vi "SessionBank.vi"(7 "Action (Get)":T1=enum."Get", 8 "error in (no error)":errorcluster, 11 "PythonSession in":refnum<class "PythonSession.lvclass">) -> (0 "error out":errorcluster, 3 "PythonSession out":refnum<class "PythonSession.lvclass">)   [LabVIEW 2022 SP3, in "PythonWrapper.lvlib" / "PythonSession.lvclass"]
uses:
  PythonSession.lvclass
  _BankAction.ctl
  PythonSession.lvclass/PythonSession.ctl
  _BankData.ctl
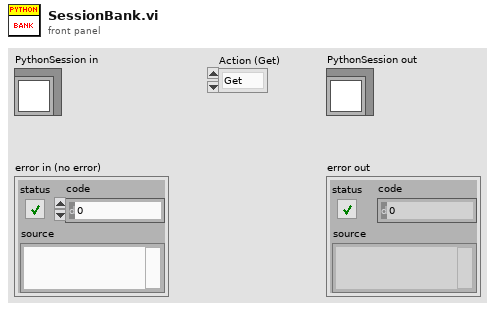
[diagram p1: front panel]
types:
  T1 = typedef "PythonWrapper.lvlib/PythonSession.lvclass/_BankAction.ctl" = enum16{"Add", "Get", "Remove"}
  T2 = typedef "PythonWrapper.lvlib/PythonSession.lvclass/_BankData.ctl" = cluster{"PythonSession":refnum<k35>, "ReferenceCounter":u32}
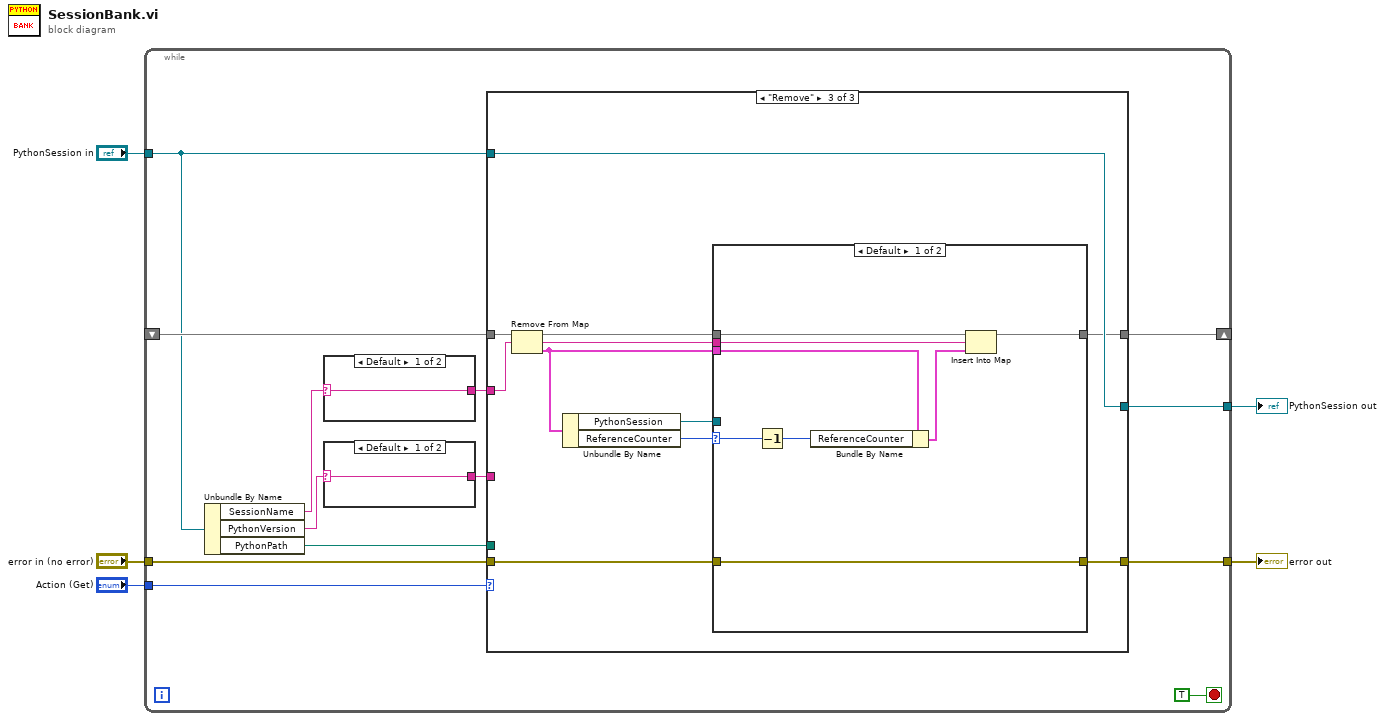
[diagram p0: block diagram]
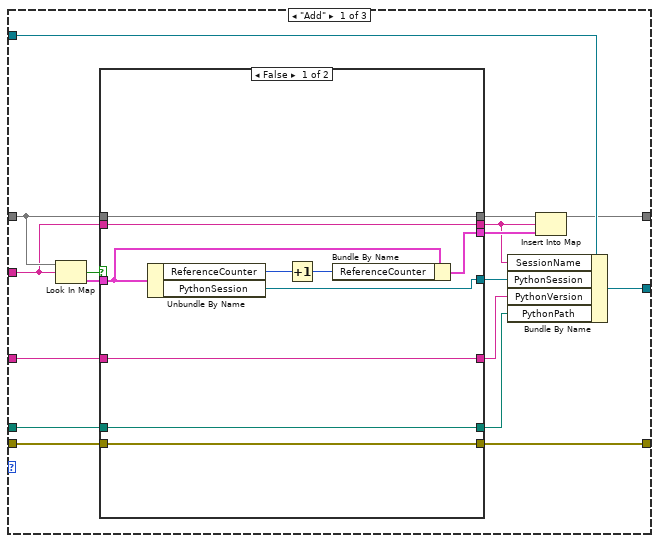
[diagram p2: hidden frame]
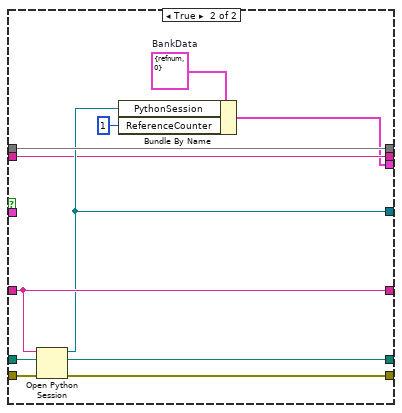
[diagram p3: hidden frame]
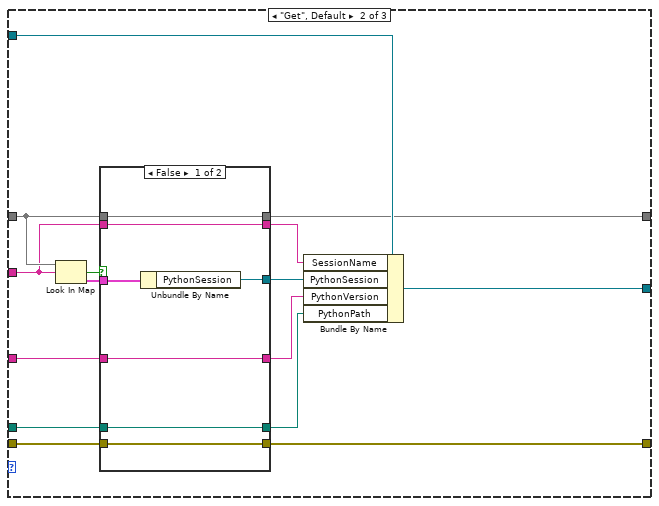
[diagram p4: hidden frame]
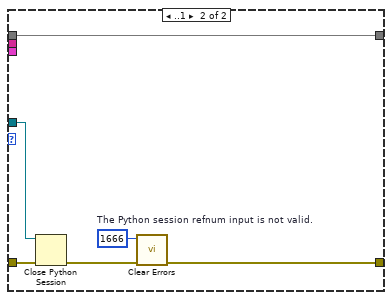
[diagram p6: hidden frame]
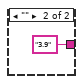
[diagram p7: hidden frame]
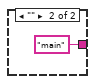
[diagram p8: hidden frame]
diagram:
  n1 = while {
    tunnel: "Action (Get)" -> [w17]
    shift-right: [w13] -> _
    shift-left: _ -> [w16]
    tunnel: "PythonSession in" -> [w10]
    tunnel: "error in (no error)" -> [w15]
    tunnel: [w14] -> w2
    tunnel: [w12] -> w1
    stop <- TRUE stop-if-true
    n2 = Unbundle By Name(w10) -> ("SessionName"=w9:string, "PythonVersion"=w7:string, "PythonPath"=w11:path)
    n3 = case shown="Default" w9 {
      selector: w9 -> [w106 _]
      tunnel: [w106 "main"] -> w8
      frame Default {
      }
      frame "" {
      }
    }
    n4 = case shown="Default" w7 {
      selector: w7 -> [w104 _]
      tunnel: [w104 "3.9"] -> w6
      frame Default {
      }
      frame "" {
      }
    }
    n5 = case shown="\"Remove\"" w17 {
      tunnel: w16 -> [w34 w69 w89]
      tunnel: w15 -> [w33 w68 w88]
      tunnel: [w32 w67 w80] -> w14
      tunnel: w6 -> [w31 w66 _]
      tunnel: w11 -> [w30 w65 _]
      tunnel: [w21 w56 w83] -> w13
      tunnel: [w27 w62 w87] -> w12
      tunnel: w10 -> [w26 w61 w87]
      tunnel: w8 -> [w25 w60 w82]
      frame "Add" {
        n6 = Look In Map(map=w34, key=w25) -> (key not found?=w35:bool, value=w29:T2)  [unwired: 1 in]
        n7 = case shown="False" w35 {
          tunnel: w34 -> [w41 w55]
          tunnel: w25 -> [w40 w48]
          tunnel: w33 -> [w45 w54]
          tunnel: [w45 w53] -> w32
          tunnel: w31 -> [w43 w51]
          tunnel: w30 -> [w44 w52]
          tunnel: [w41 w55] -> w22
          tunnel: w29 -> [w39 _]
          tunnel: [w42 w49] -> w28
          tunnel: [w44 w52] -> w24
          tunnel: [w43 w51] -> w23
          tunnel: [w40 w48] -> w19
          tunnel: [w37 w47] -> w20
          frame False {
            n8 = Unbundle By Name(w39) -> ("ReferenceCounter"=w36:u32, "PythonSession"=w42:refnum<k35>)
            n9 = Increment(x=w36) -> (x+1=w38:u32)
            n10 = Bundle By Name(cluster=w39, "ReferenceCounter"=w38) -> (w37:T2)
          }
          frame True {
            w50 = T2 {"PythonSession"=refnum, "ReferenceCounter"=0}  # BankData
            n11 = Open Python Session(python version=w51, python path=w52, 3:w54) -> (session out=w49:refnum<k35>, error out=w53:errorcluster)
            n12 = Bundle By Name(cluster=w50, "PythonSession"=w49, "ReferenceCounter"=u32 1) -> (w47:T2)
          }
        }
        n13 = Bundle By Name(cluster=w26, "SessionName"=w19, "PythonSession"=w28, "PythonVersion"=w23, "PythonPath"=w24) -> (w27:refnum<class "PythonSession.lvclass">)
        n14 = Insert Into Map(map in=w22, key=w19, value=w20) -> (map out=w21:map{string, T2})  [unwired: 2 out]
      }
      frame "Get", Default {
        n15 = Look In Map(map=w69, key=w60) -> (key not found?=w70:bool, value=w64:T2)  [unwired: 1 in]
        n16 = case shown="False" w70 {
          tunnel: w69 -> [w72 w79]
          tunnel: w60 -> [w71 _]
          tunnel: w68 -> [w77 w78]
          tunnel: [w77 w78] -> w67
          tunnel: w66 -> [w75 _]
          tunnel: w65 -> [w76 _]
          tunnel: [w72 w79] -> w56
          tunnel: w64 -> [w73 _]
          tunnel: [w74 _] -> w63
          tunnel: [w76 _] -> w59
          tunnel: [w75 _] -> w58
          tunnel: [w71 _] -> w57
          frame False {
            n17 = Unbundle By Name(w73) -> ("PythonSession"=w74:refnum<k35>)
          }
          frame True {
          }
        }
        n18 = Bundle By Name(cluster=w61, "SessionName"=w57, "PythonSession"=w63, "PythonVersion"=w58, "PythonPath"=w59) -> (w62:refnum<class "PythonSession.lvclass">)
      }
      frame "Remove" {
        n19 = Remove From Map(10:w82, 11:w89) -> (1:w81:T2, 3:w84:map{string, T2})  [unwired: 1 out]
        n20 = Unbundle By Name(w81) -> ("PythonSession"=w85:refnum<k35>, "ReferenceCounter"=w86:u32)
        n21 = case shown="Default" w86 {
          selector: w86 -> [w92 _]
          tunnel: w88 -> [w96 w103]
          tunnel: [w96 w98] -> w80
          tunnel: w85 -> [_ w102]
          tunnel: w84 -> [w97 w101]
          tunnel: [w95 w101] -> w83
          tunnel: w82 -> [w94 _]
          tunnel: w81 -> [w93 _]
          frame Default {
            n22 = Decrement(x=w92) -> (x-1=w91:u32)
            n23 = Bundle By Name(cluster=w93, "ReferenceCounter"=w91) -> (w90:T2)
            n24 = Insert Into Map(map in=w97, key=w94, value=w90) -> (map out=w95:map{string, T2})  [unwired: 2 out]
          }
          frame ..1 {
            w99 = 1666  # The Python session refnum input is not valid.
            n25 = Close Python Session(session in=w102, error in=w103) -> (11:w100:errorcluster)
            n26 = call <vilib>:"Clear Errors.vi"("error in (no error)"=w100, "specific error code to clear (0: all)"=w99) -> ("error out"=w98:errorcluster)  [unwired: 4 in, 1 out]
          }
        }
      }
    }
  }
  "PythonSession out" <- w1
  "error out" <- w2
